vi "libdaq_dac_start.vi"(0 "error in (no error)":errorcluster, 1 "device_name":string, 2 "module_name":string) -> (14 "error out":errorcluster, 15 "device_name":string, 16 "module_name":string)   [LabVIEW 2010, in "libdaqVI.lvlib"]
doc: "触发DAC模块输出，只对DAC_TRIGGER_MODE_SOFT模式有效"
uses:
  libdaqVI.lvlib
  dll/daqlib.dll
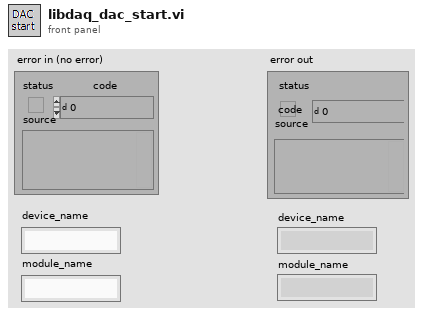
[diagram p1: front panel]
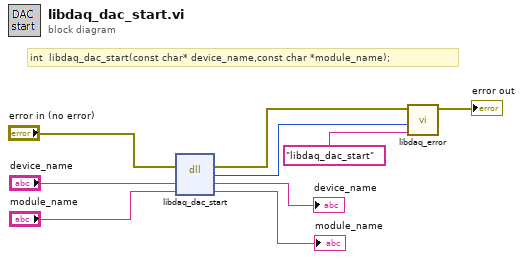
[diagram p0: block diagram]
diagram:
  # "int  libdaq_dac_start(const char* device_name,const char *module_name);"
  n1 = dll-call lib="E:/Product/Example/DAQ-USB3212/Labview/labview_2010/libdaqVI/dll/daqlib.dll" fn="libdaq_dac_start"(error in="error in (no error)", "device_name"="device_name", "module_name"="module_name") -> (error out=w7:errorcluster, "return type"=w5:i32, "device_name"=→"device_name":string, "module_name"=→"module_name":string)  [unwired: 2 in, 1 out]
  n2 = call "libdaq_error.vi"("error source"="libdaq_dac_start", "error code"=w5, "错误输入（无错误）"=w7) -> ("错误输出"=→"error out":errorcluster)  [unwired: 8 in]
